vi "Config Display.vi"(0 "VISA resource name":refnum<visa-resource-name>, 5 "Channel (1: CH1)":u16(ring)=1 items=["", "CH1", "CH2", "CH3", "CH4", "CH5", "CH6", "CH7", "CH8"], 7 "Display (F: OFF)":bool, 11 "error in (no error)":errorcluster) -> (4 "VISA resource name out":refnum<visa-resource-name>, 15 "error out":errorcluster)   [LabVIEW 2013, in "Yokogawa.lvlib" / "Yokogawa PZ4000.lvlib"]
doc: "This VI sends the Display group command to the PZ4000 series."
uses:
  Yokogawa PZ4000.lvlib
panel:
  # "ON\nOFF"
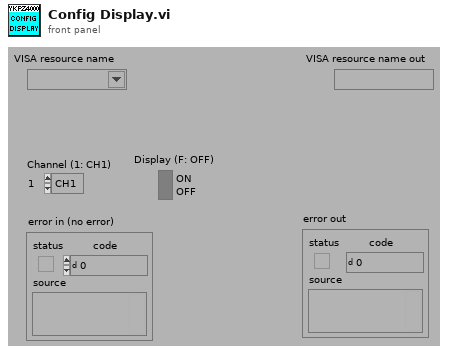
[diagram p1: front panel]
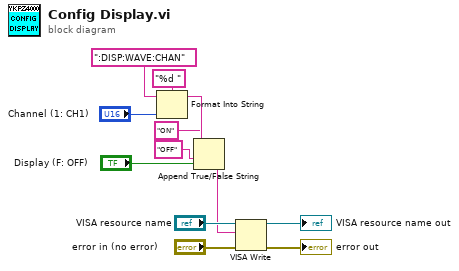
[diagram p0: block diagram]
diagram:
  n1 = Format Into String(format string="%d ", initial string=":DISP:WAVE:CHAN", "Channel (1: CH1)") -> (resulting string=w8:string)  [unwired: 1 in, 1 out]
  n2 = Append True/False String(1:"Display (F: OFF)", 2:"OFF", 3:"ON", 4:w8) -> (0:w2:string)
  n3 = VISA Write(VISA resource name="VISA resource name", write buffer=w2, error in (no error)="error in (no error)") -> (VISA resource name out=→"VISA resource name out":refnum<visa-resource-name>, error out=→"error out":errorcluster)  [unwired: 1 out]
